vi "PAN_DBS_AddAsSTR.vi"(9 "offset":string, 10 "ini value":string) -> (1 "ok?":bool, 2 "value out":string)   [LabVIEW 2016]
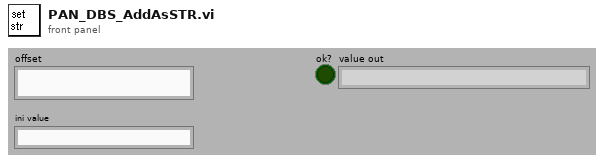
[diagram p1: front panel]
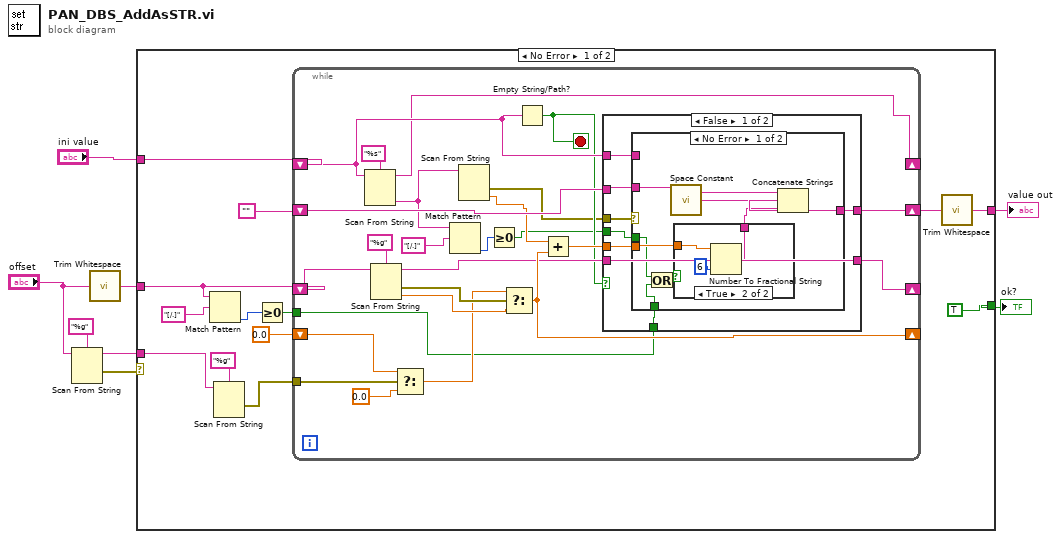
[diagram p0: block diagram]
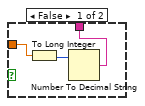
[diagram p2: hidden frame]
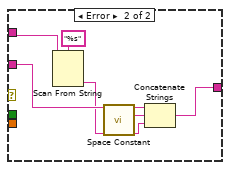
[diagram p3: hidden frame]
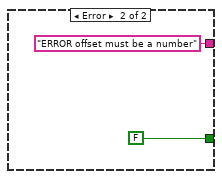
[diagram p5: hidden frame]
diagram:
  n1 = Scan From String(format string="%g", input string="offset") -> (remaining string=w2:string, error out=w5:errorcluster)  [unwired: 2 in, 3 out]
  n2 = call <vilib>:"Trim Whitespace.vi"("string"="offset") -> ("trimmed string"=w1:string)  [unwired: 1 in]
  n3 = case shown="No Error" w5 {
    tunnel: "ini value" -> [w21 _]
    tunnel: w1 -> [w12 _]
    tunnel: [TRUE ("set?") FALSE ("set?")] -> w4
    tunnel: [w16 "ERROR offset must be a number"] -> w3
    tunnel: w2 -> [w14 _]
    frame No Error {
      n4 = Match Pattern(string=w12, regular expression="[/.]") -> (offset past match=w11:i32)  [unwired: 4 out]
      n5 = Scan From String(format string="%g", input string=w14) -> (error out=w13:errorcluster)  [unwired: 2 in, 4 out]
      n6 = Greater Or Equal To 0?(x=w11) -> (x >= 0?=w10:bool)
      n7 = while {
        shift-right: [w34] -> _
        shift-left: w21 -> [w35]
        shift-right: [w37] -> _
        shift-left: w12 -> [w44]
        shift-right: [w42] -> w19
        shift-left: "" -> [w41]
        shift-right: [w39] -> _
        shift-left: 0.0 -> [w28]
        tunnel: w13 -> [w30]
        tunnel: w10 -> [w26]
        stop <- w33 stop-if-true
        n8 = Scan From String(format string="%s", input string=w35) -> (remaining string=w34:string, output 1=w24:string)  [unwired: 2 in, 3 out]
        n9 = Scan From String(format string="%g", input string=w44) -> (remaining string=w38:string, error out=w36:errorcluster, output 1=w40:dbl)  [unwired: 2 in, 2 out]
        n10 = Select(t=w28, s=w30, f=0.0 ("t")) -> (s? t:f=w29:dbl)
        n11 = Match Pattern(string=w24, regular expression="[/.]") -> (offset past match=w23:i32)  [unwired: 4 out]
        n12 = Scan From String(input string=w24) -> (error out=w31:errorcluster, output 1=w32:dbl)  [unwired: 3 in, 3 out]
        n13 = Greater Or Equal To 0?(x=w23) -> (x >= 0?=w22:bool)
        n14 = Select(t=w29, s=w36, f=w40) -> (s? t:f=w39:dbl)
        n15 = Empty String/Path?(string/path=w35) -> (empty?=w33:bool)
        n16 = Add(x=w32, y=w39) -> (x+y=w43:dbl)
        n17 = case shown="False" w33 {
          tunnel: w43 -> [w54 _]
          tunnel: [w53 w76] -> w42
          tunnel: w41 -> [w52 w76]
          tunnel: w38 -> [w51 w75]
          tunnel: [w51 w75] -> w37
          tunnel: w31 -> [w50 _]
          tunnel: w35 -> [w49 _]
          tunnel: w26 -> [w48 _]
          tunnel: w22 -> [w47 _]
          frame False {
            n18 = case shown="No Error" w50 {
              tunnel: w54 -> [w59 _]
              tunnel: [w62 w69] -> w53
              tunnel: w52 -> [w60 w71]
              tunnel: w49 -> [_ w74]
              tunnel: w48 -> [w56 _]
              tunnel: w47 -> [w55 _]
              frame No Error {
                n19 = Or(x=w55, y=w56) -> (x .or. y?=w57:bool)
                n20 = call <vilib>:"Space Constant.vi"() -> ("String"=w61:string)
                n21 = case shown="True" w57 {
                  tunnel: w59 -> [w65 w68]
                  tunnel: [w63 w66] -> w58
                  frame False {
                    n22 = To Long Integer(number=w65) -> (32bit integer=w64:i32)
                    n23 = Number To Decimal String(number=w64) -> (decimal integer string=w63:string)  [unwired: 1 out]
                  }
                  frame True {
                    n24 = Number To Fractional String(number=w68, precision (6)=i16 6) -> (F-format string=w66:string)  [unwired: 2 out]
                  }
                }
                n25 = Concatenate Strings(w60, w61, w58) -> (w62:string)
              }
              frame Error {
                n26 = Scan From String(format string="%s", input string=w74) -> (output 1=w70:string)  [unwired: 2 in, 4 out]
                n27 = call <vilib>:"Space Constant.vi"() -> ("String"=w72:string)
                n28 = Concatenate Strings(w71, w72, w70) -> (w69:string)
              }
            }
          }
          frame True {
          }
        }
      }
      n29 = call <vilib>:"Trim Whitespace.vi"("string"=w19) -> ("trimmed string"=w16:string)  [unwired: 1 in]
    }
    frame Error {
    }
  }
  "ok?" <- w4
  "value out" <- w3
